vi "verify unique parameter in range - SET.vi"(8 "error in (no error)":errorcluster, 9 "value":dbl, 10 "parameter name":string, 11 "Simulated_CCD_Camera in":refnum<class "Simulated Camera.lvclass">) -> (0 "error out":errorcluster, 3 "Simulated_CCD_Camera out":refnum<class "Simulated Camera.lvclass">)   [LabVIEW 2018, in "Simulated Camera.lvclass"]
uses:
  Simulated Camera.lvclass
  Simulated Camera.lvclass/Simulated Camera.ctl
  <vilib>/ErrorRing/Error Ring.xnode
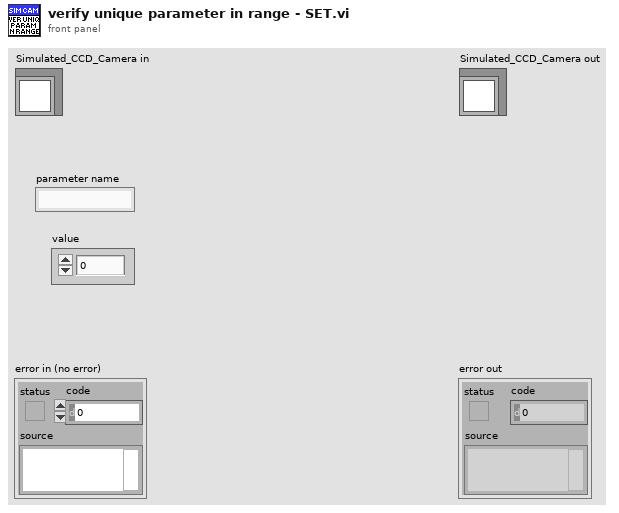
[diagram p1: front panel]
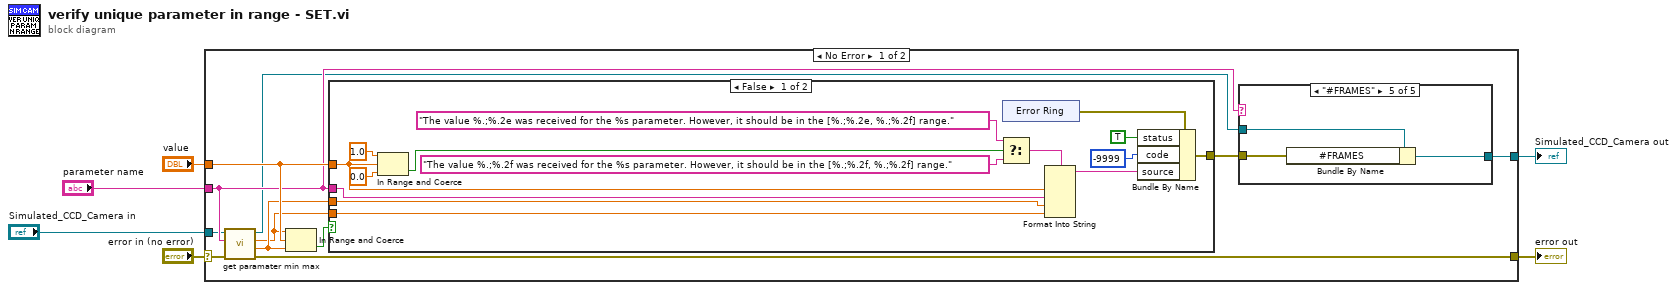
[diagram p0: block diagram]
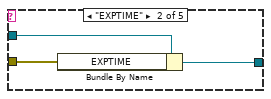
[diagram p3: hidden frame]
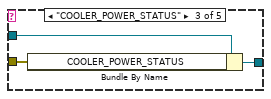
[diagram p4: hidden frame]
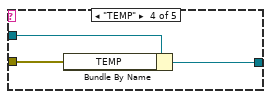
[diagram p5: hidden frame]
diagram:
  n1 = case shown="No Error" "error in (no error)" {
    selector: "error in (no error)" -> [w11 w48]
    tunnel: [w7 w48] -> w5
    tunnel: [w8 w47] -> w4
    tunnel: "Simulated_CCD_Camera in" -> [w12 w47]
    tunnel: "value" -> [w16 _]
    tunnel: "parameter name" -> [w15 _]
    frame No Error {
      n2 = call "get paramater min max.vi"("error in (no error)"=w11, "parameter name"=w15, "Simulated Camera in"=w12) -> ("error out"=w7:errorcluster, "min"=w14:dbl, "max"=w13:dbl, "Simulated Camera out"=w10:refnum<class "Simulated Camera.lvclass">)  [unwired: 5 in]
      n3 = In Range and Coerce(upper limit=w13, x=w16, lower limit=w14) -> (In Range?=w17:bool)  [unwired: 1 out]
      n4 = case shown="False" w17 {
        tunnel: w15 -> [w32 _]
        tunnel: w16 -> [w37 _]
        tunnel: w14 -> [w41 _]
        tunnel: w13 -> [w40 _]
        tunnel: [w31 _] -> w9
        frame False {
          n5 = In Range and Coerce(upper limit=1.0, x=w37, lower limit=0.0 ("upper limit")) -> (In Range?=w36:bool)  [unwired: 1 out]
          n6 = Select(t="The value %.;%.2e was received for the %s parameter. However, it should be in the [%.;%.2e, %.;%.2f] range." ("string"), s=w36, f="The value %.;%.2f was received for the %s parameter. However, it should be in the [%.;%.2f, %.;%.2f] range." ("string")) -> (s? t:f=w33:string)
          n7 = xnode "Error Ring"() -> ("error out"=w45:errorcluster)
          n8 = Format Into String(format string=w33, w37, w32, w41, w40) -> (resulting string=w42:string)  [unwired: 2 in, 1 out]
          n9 = Bundle By Name(cluster=w45, "status"=TRUE, "code"=-9999, "source"=w42) -> (w31:errorcluster)
        }
        frame True {
        }
      }
      n10 = case shown="\"#FRAMES\"" w15 {
        tunnel: w10 -> [w18 w21 w24 w27 w30]
        tunnel: [w18 w20 w23 w26 w29] -> w8
        tunnel: w9 -> [_ w19 w22 w25 w28]
        frame "False", Default {
        }
        frame "EXPTIME" {
          n11 = Bundle By Name(cluster=w21, "EXPTIME"=w19) -> (w20:refnum<class "Simulated Camera.lvclass">)
        }
        frame "COOLER_POWER_STATUS" {
          n12 = Bundle By Name(cluster=w24, "COOLER_POWER_STATUS"=w22) -> (w23:refnum<class "Simulated Camera.lvclass">)
        }
        frame "TEMP" {
          n13 = Bundle By Name(cluster=w27, "TEMP"=w25) -> (w26:refnum<class "Simulated Camera.lvclass">)
        }
        frame "#FRAMES" {
          n14 = Bundle By Name(cluster=w30, "#FRAMES"=w28) -> (w29:refnum<class "Simulated Camera.lvclass">)
        }
      }
    }
    frame Error {
    }
  }
  "error out" <- w5
  "Simulated_CCD_Camera out" <- w4
